vi "TX example.vi"() -> ()   [LabVIEW 2016]
uses:
  <vilib>/Analysis/NI_AALPro.lvlib
  <vilib>/Analysis/2dsp.llb/Complex FFT.vi
panel:
  out "S(t)":dbl[](graph)
  out "S(w)":dbl[](graph)
  in  "CarrierFreqHz":dbl(slide)=90658509.45494995 scale=86000000.0..110000000.0 scale format="%#_6p"
  in  "VGAGainDb":dbl=20.0 min=0.0 max=62.0 step=2.0
  in  "stop":bool
  in  "SampleFreqHz":dbl=4500000.0 format="%#_6p"
  in  "FilterBandwidthHz":dbl=3000000.0 format="%#_6p"
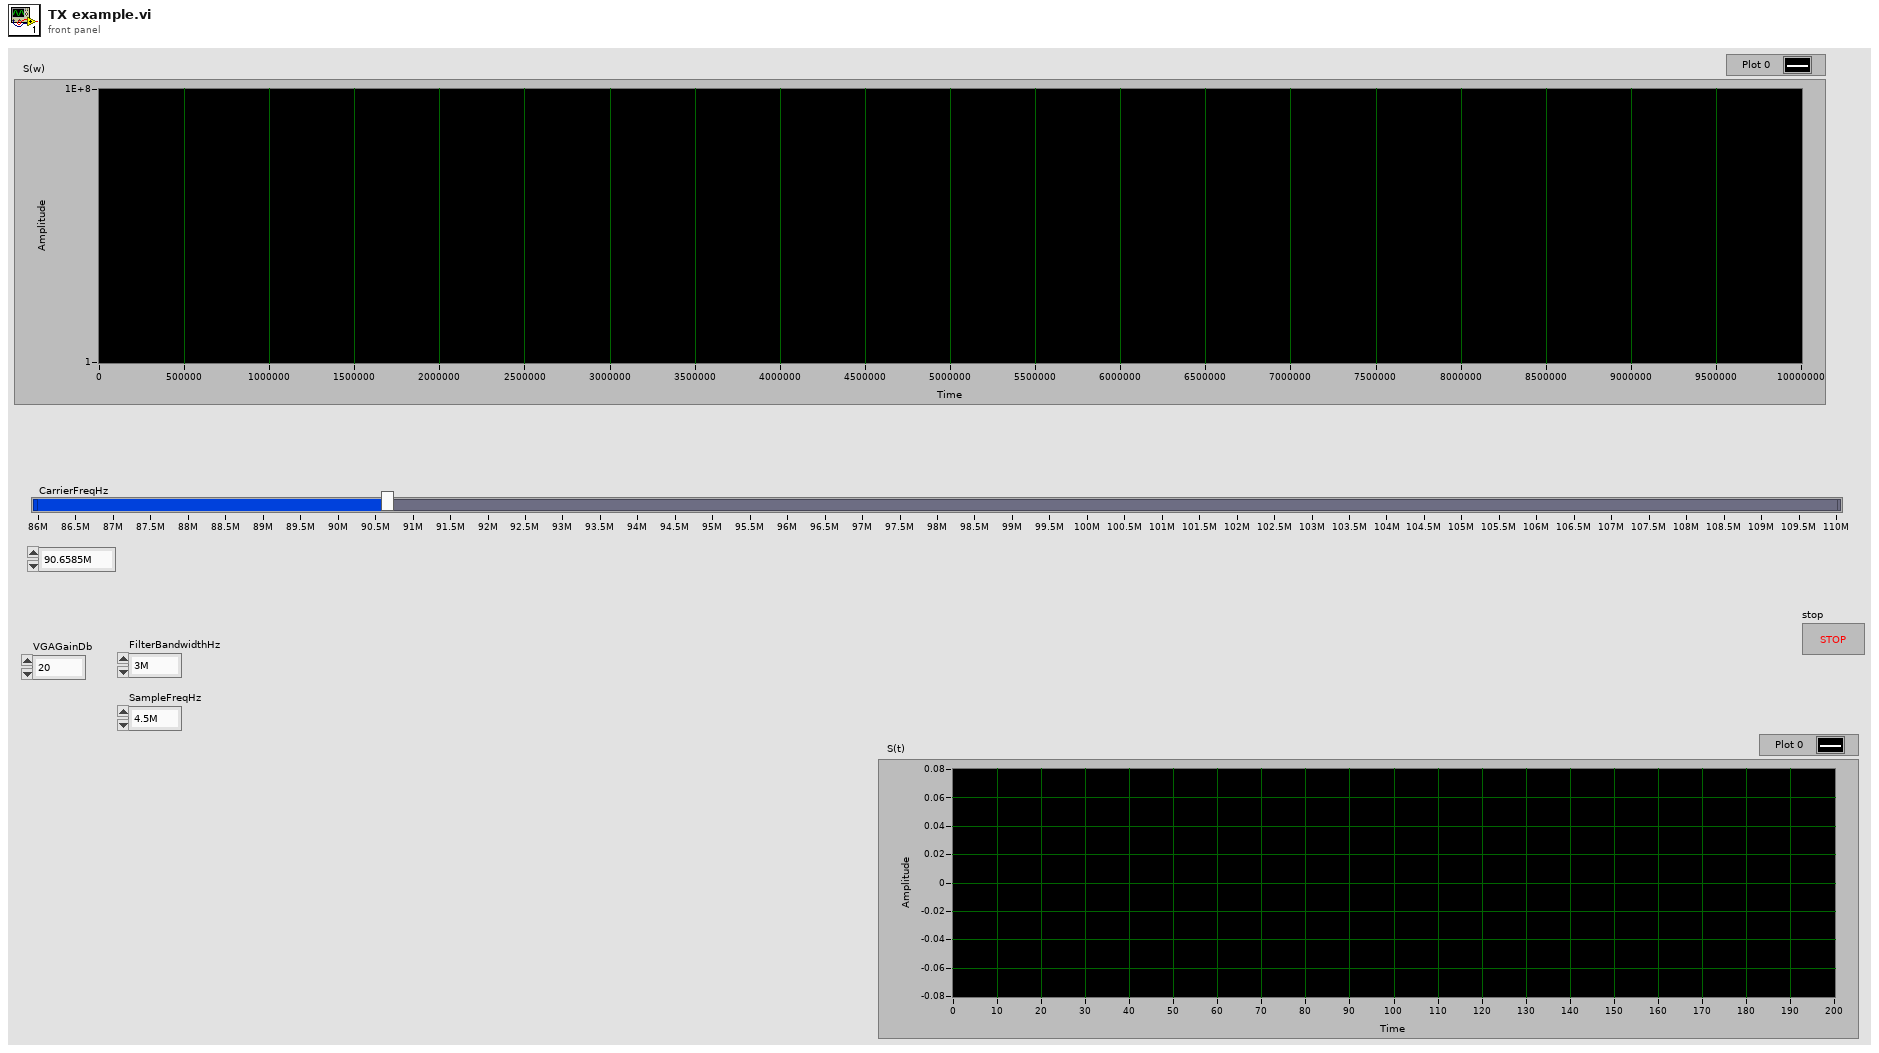
[diagram p1: front panel]
types:
  T1 = typedef "HackRF_Ref.ctl" = cluster{".net":refnum<k24>, "HackrfDeviceList":refnum<k24>[], "OpenDevice":refnum<k24>, "StartRX":refnum<k24>, "CarrierFreqHz":dbl, "SampleFreqHz":dbl, "FilterBandwidthHz":dbl, "AMPEnable":bool, "LNAGainDb":dbl, "VGAGainDb":dbl, "StartTx":refnum<k24>}
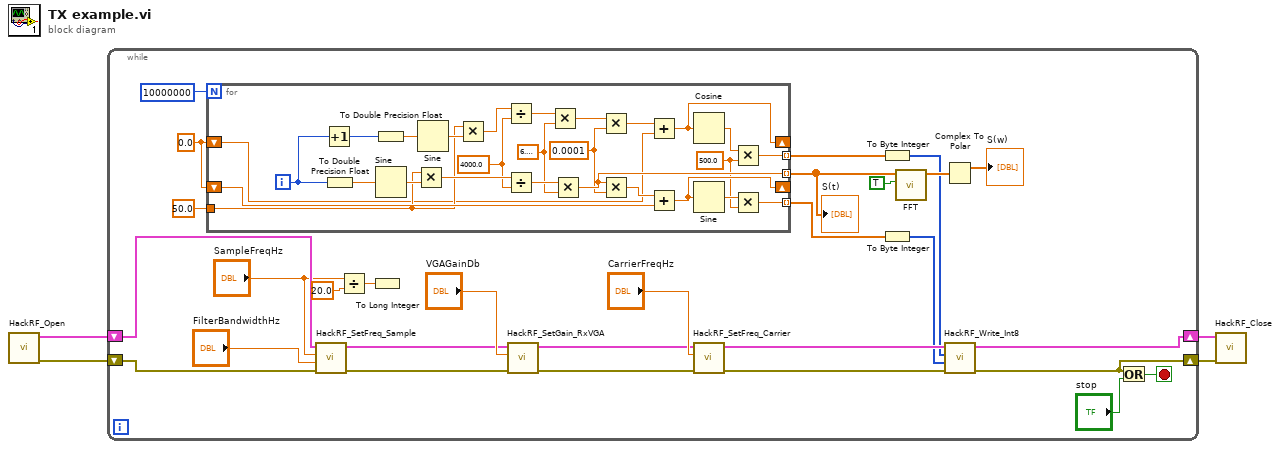
[diagram p0: block diagram]
diagram:
  n1 = call "HackRF_Open.vi"() -> ("error out"=w3:errorcluster, "Cluster"=w4:T1)  [unwired: 10 in]
  n2 = while {
    shift-right: [w19] -> w2
    shift-left: w4 -> [w33]
    shift-right: [w18] -> w1
    shift-left: w3 -> [w32]
    stop <- w23 stop-if-true
    w15 = 0.0
    n3 = for {
      N: 10000000 -> [_]
      tunnel: 50.0 -> [w46]
      shift-right: [w52] -> _
      shift-left: w15 -> [w56]
      tunnel: [w55] -> w9 mode=indexing
      tunnel: [w51] -> w5 mode=indexing
      shift-right: [w39] -> _
      shift-left: w15 -> [w41]
      tunnel: [w38] -> w6 mode=indexing
      i -> [w50]
      w37 = 500.0 ("y")
      w36 = 0.0001 ("y")
      w35 = 6.283185307179586
      w34 = 4000.0 ("y")
      n4 = Increment(x=w50) -> (x+1=w48:i32)
      n5 = To Double Precision Float(number=w50) -> (double precision float=w60:dbl)
      n6 = To Double Precision Float(number=w48) -> (double precision float=w49:dbl)
      n7 = Sine(x=w60) -> (sin(x)=w59:dbl)
      n8 = Multiply(x=w46, y=w59) -> (x*y=w58:dbl)
      n9 = Sine(x=w49) -> (sin(x)=w47:dbl)
      n10 = Multiply(x=w46, y=w47) -> (x*y=w45:dbl)
      n11 = Divide(x=w45, y=w34) -> (x/y=w44:dbl)
      n12 = Divide(x=w58, y=w34) -> (x/y=w57:dbl)
      n13 = Multiply(x=w44, y=w35) -> (x*y=w43:dbl)
      n14 = Multiply(x=w57, y=w35) -> (x*y=w55:dbl)
      n15 = Multiply(x=w43, y=w36) -> (x*y=w42:dbl)
      n16 = Multiply(x=w55, y=w36) -> (x*y=w54:dbl)
      n17 = Add(x=w42, y=w41) -> (x+y=w39:dbl)
      n18 = Add(x=w54, y=w56) -> (x+y=w52:dbl)
      n19 = Cosine(x=w39) -> (cos(x)=w40:dbl)
      n20 = Sine(x=w52) -> (sin(x)=w53:dbl)
      n21 = Multiply(x=w40, y=w37) -> (x*y=w38:dbl)
      n22 = Multiply(x=w53, y=w37) -> (x*y=w51:dbl)
    }
    "S(t)" <- w9
    n23 = call "HackRF_SetFreq_Sample.vi"("error in (no error)"=w32, "FilterBandwidthHz"="FilterBandwidthHz", "SampleFreqHz"="SampleFreqHz", "HackRF in"=w33) -> ("error out"=w12:errorcluster, "HackRF out"=w13:T1)  [unwired: 6 in]
    n24 = Divide(x="SampleFreqHz", y=20.0) -> (x/y=w29:dbl)
    n25 = To Long Integer(number=w29) -> ()  [unwired: 1 out]
    n26 = call "HackRF_SetGain_RxVGA.vi"("error in (no error)"=w12, "VGAGainDb"="VGAGainDb", "HackRF in"=w13) -> ("error out"=w10:errorcluster, "HackRF out"=w11:T1)  [unwired: 7 in]
    n27 = call "HackRF_SetFreq_Carrier.vi"("error in (no error)"=w10, "CarrierFreqHz"="CarrierFreqHz", "HackRF_In"=w11) -> ("error out"=w20:errorcluster, "HackRF_Out"=w21:T1)  [unwired: 7 in]
    n28 = To Byte Integer(number=w6) -> (8bit integer=w8:i8[])
    n29 = To Byte Integer(number=w5) -> (8bit integer=w7:i8[])
    n30 = call-poly <vilib>:"FFT.vi"("shift?"=TRUE, "X"=w9) -> ("FFT {X}"=w25:cdb[])  [unwired: 8 in, 1 out]
    n31 = Complex To Polar(r * e^(i*theta)=w25) -> (r=→"S(w)":dbl[])  [unwired: 1 out]
    n32 = call "HackRF_Write_Int8.vi"("error in (no error)"=w20, "Q data"=w7, "I data"=w8, "HackRF"=w21) -> ("error out"=w18:errorcluster, "HackRF"=w19:T1)  [unwired: 6 in]
    n33 = Or(x=w18, y="stop") -> (x .or. y?=w23:bool)
  }
  n34 = call "HackRF_Close.vi"("error in (no error)"=w1, "Cluster in"=w2) -> ()  [unwired: 8 in, 2 out]
